vi "Quinn's First Interpolation method.vi"(8 "FFT array Im":dbl[](array[numeric]), 11 "FFT array Re":dbl[](array[numeric])) -> (0 "max index(es)":i32, 3 "Index Bin":dbl)   [LabVIEW 2014]
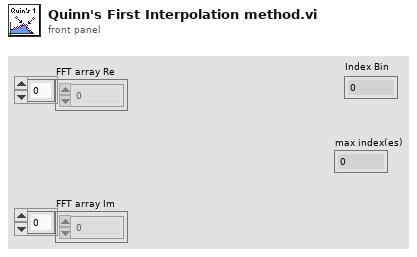
[diagram p1: front panel]
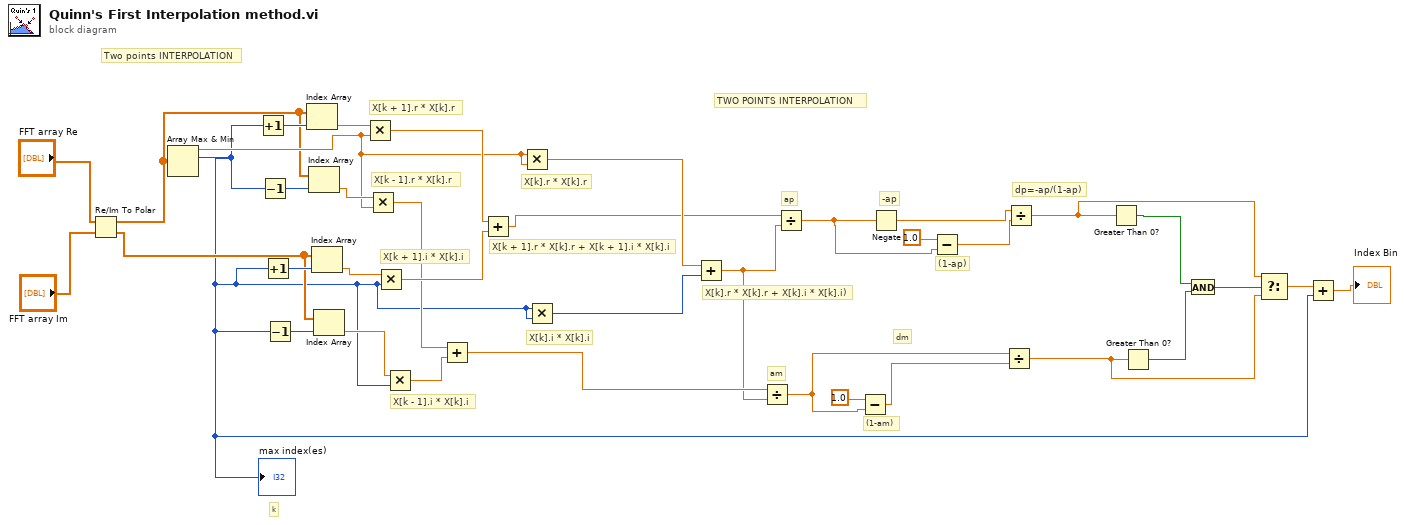
[diagram p0: block diagram]
diagram:
  # "TWO POINTS INTERPOLATION"
  # "Two points INTERPOLATION"
  # "k"
  # "dm"
  # "(1-am)"
  # "am"
  # "X[k - 1].r * X[k].r"
  # "X[k - 1].i * X[k].i"
  # "dp=-ap/(1-ap)"
  # "(1-ap)"
  # "-ap"
  # "ap"
  # "X[k].r * X[k].r + X[k].i * X[k].i)"
  # "X[k + 1].r * X[k].r + X[k + 1].i * X[k].i"
  # "X[k].r * X[k].r"
  # "X[k].i * X[k].i"
  # "X[k + 1].i * X[k].i"
  # "X[k + 1].r * X[k].r"
  n1 = Re/Im To Polar(2:"FFT array Im", 3:"FFT array Re") -> (0:w3:dbl[], 1:w4:dbl[])
  n2 = Array Max & Min(array=w4) -> (max value=w20:dbl, max index (indices)=w2:i32)  [unwired: 2 out]
  "max index(es)" <- w2
  n3 = Increment(x=w2) -> (x+1=w37:i32)
  n4 = Decrement(x=w2) -> (x-1=w36:i32)
  n5 = Increment(x=w2) -> (x+1=w34:i32)
  n6 = Decrement(x=w2) -> (x-1=w35:i32)
  n7 = Index Array(array=w4, index=w37) -> (element=w33:dbl)
  n8 = Index Array(array=w4, index=w36) -> (element=w21:dbl)
  n9 = Index Array(array=w3, index=w34) -> (element=w32:dbl)
  n10 = Index Array(array=w3, index=w35) -> (element=w22:dbl)
  n11 = Multiply(x=w33, y=w20) -> (x*y=w31:dbl)
  n12 = Multiply(x=w21, y=w20) -> (x*y=w18:dbl)
  n13 = Multiply(x=w32, y=w2) -> (x*y=w30:dbl)
  n14 = Multiply(x=w22, y=w2) -> (x*y=w19:dbl)
  n15 = Add(x=w18, y=w19) -> (x+y=w17:dbl)
  n16 = Add(x=w31, y=w30) -> (x+y=w27:dbl)
  n17 = Multiply(x=w20, y=w20) -> (x*y=w28:dbl)
  n18 = Multiply(x=w2, y=w2) -> (x*y=w29:i32)
  n19 = Add(x=w28, y=w29) -> (x+y=w16:dbl)
  n20 = Divide(x=w17, y=w16) -> (x/y=w14:dbl)
  n21 = Divide(x=w27, y=w16) -> (x/y=w25:dbl)
  n22 = Subtract(x=1.0, y=w14) -> (x-y=w13:dbl)
  n23 = Negate(x=w25) -> (-x=w24:dbl)
  n24 = Subtract(x=1.0, y=w25) -> (x-y=w23:dbl)
  n25 = Divide(x=w14, y=w13) -> (x/y=w8:dbl)
  n26 = Divide(x=w24, y=w23) -> (x/y=w9:dbl)
  n27 = Greater Than 0?(x=w9) -> (x > 0?=w11:bool)
  n28 = Greater Than 0?(x=w8) -> (x > 0?=w12:bool)
  n29 = And(x=w11, y=w12) -> (x .and. y?=w10:bool)
  n30 = Select(t=w9, s=w10, f=w8) -> (s? t:f=w7:dbl)
  n31 = Add(x=w7, y=w2) -> (x+y=→"Index Bin":dbl)
